vi "LaunchVI.vi"(8 "Error In":errorcluster, 11 "Name":string) -> (0 "Error Out":errorcluster)   [LabVIEW 2018]
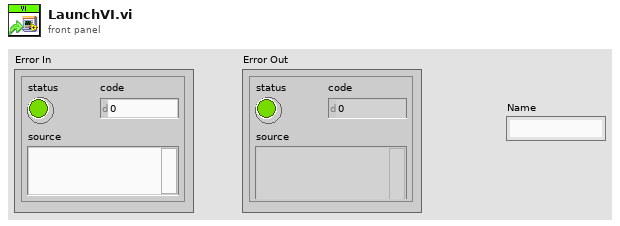
[diagram p1: front panel]
types:
  T1 = enum16{"Always On", "Always Off", "Off While Running"}
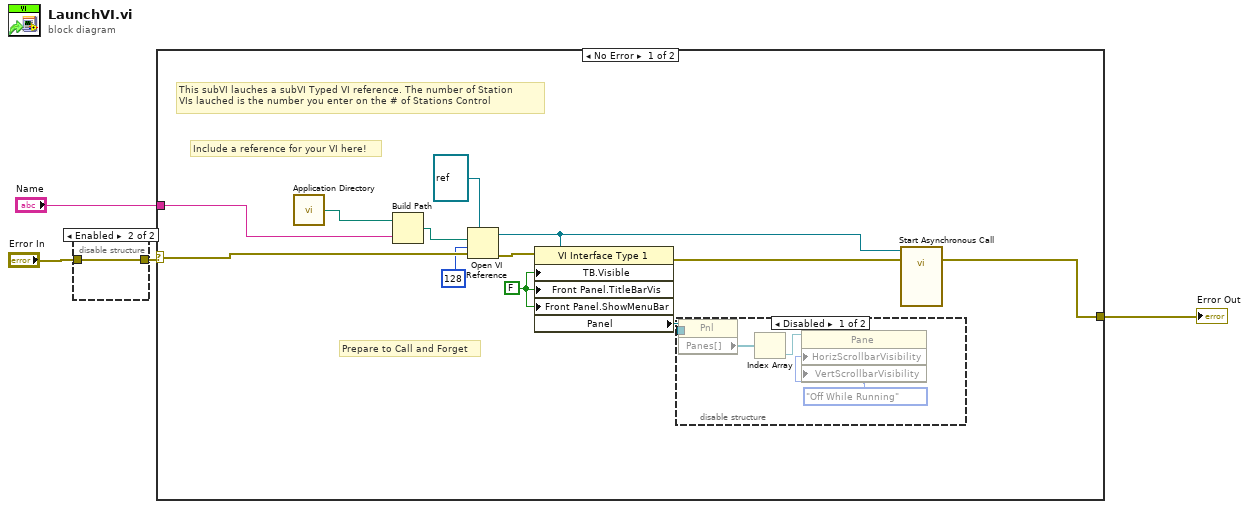
[diagram p0: block diagram]
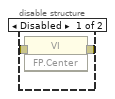
[diagram p2: hidden frame]
diagram:
  n1 = disable-structure shown="Enabled" {
    disable-tunnel: [w6 w7] -> w3
    disable-tunnel: "Error In" -> [w5 w7]
    frame Disabled {
      n2 = invoke class="VI" method="FP.Center"(error in=w5) -> (error out=w6:errorcluster)  [unwired: 2 in, 2 out]
    }
    frame Enabled {
    }
  }
  n3 = case shown="No Error" w3 {
    selector: w3 -> [w18 w24]
    tunnel: [w19 w24] -> w4
    tunnel: "Name" -> [w11 _]
    frame No Error {
      w15 = FALSE
      # "Include a reference for your VI here!"
      # "Prepare to Call and Forget"
      # "This subVI lauches a subVI Typed VI reference. The number of Station\nVIs lauched is the number you enter on the # of Stations Control"
      n4 = call <vilib>:"Application Directory.vi"() -> ("Application Directory"=w10:path)
      n5 = Build Path(base path=w10, name or relative path=w11) -> (appended path=w9:path)
      n6 = Open VI Reference(type specifier VI Refnum (for type only)=refnum<vi> refnum, vi path=w9, options=128, error in (no error)=w18) -> (vi reference=w12:refnum<vi>, error out=w14:errorcluster)  [unwired: 2 in]
      n7 = property class="VI Interface Type 1"(reference=w12, error in=w14, "TB.Visible"=w15, "Front Panel.TitleBarVis"=w15, "Front Panel.ShowMenuBar"=w15) -> (error out=w13:errorcluster, "Panel"=w16:refnum<vi>)  [unwired: 1 out]
      n8 = disable-structure shown="Disabled" {
        disable-tunnel: w16 -> [w23 _]
        frame Disabled {
          w20 = T1."Off While Running" ("Horizontal Scrollbar Visibility")
          n9 = property class="Pnl"(reference=w23) -> ("Panes[]"=w21:refnum<vi>[])  [unwired: 1 in, 2 out]
          n10 = Index Array(array=w21) -> (element=w22:refnum<vi>)  [unwired: 1 in]
          n11 = property class="Pane"(reference=w22, "HorizScrollbarVisibility"=w20, "VertScrollbarVisibility"=w20) -> ()  [unwired: 1 in, 2 out]
        }
        frame Enabled {
        }
      }
      n12 = call-by-ref "Start Asynchronous Call"(reference=w12, error in=w13) -> (error out=w19:errorcluster)  [unwired: 12 in, 1 out]
    }
    frame Error {
      # "In case an error is entered in this SubVI, no code is executed and the error is propagated."
    }
  }
  "Error Out" <- w4
